vi "Behaviour Tree.vi"(10 "IO":T1) -> (3 "bt_Node out":refnum<class "bt_Node.lvclass">)   [LabVIEW 2021, in "Car Wash Support.lvlib"]
uses:
  Car Wash Support.lvlib
  IO Refs.ctl
  <vilib>/TSA/Abstract Data Classes/Abs_Types/Boolean/Abs_Boolean.lvclass
  <vilib>/TSA/Abstract Data Classes/Abs_Types/I32 Integer/Abs_I32 Integer.lvclass
  <vilib>/TSA/Abstract Data Classes/Abs_Types/Double Float/Abs_Double Float.lvclass
  <vilib>/TSA/Event Log/Event_TextLog/Event_TextLog.lvclass
  C:/Program Files (x86)/National Instruments/LabVIEW 2021/vi.lib/TSA/Event Log/abs_EventLog/abs_EventLog.lvclass
  Wash Indicators.ctl
  Wash Options.ctl
  Support/Nodes/abs_Node/bt_Node.lvclass
  Support/Nodes/Decorators/Repeater/Support/Finish On - Type.ctl
  Support/Nodes/Leaves/Log/bt_Log.lvclass
  C:/Users/timst/Documents/Repositories/LV_Behaviour_Tree/Source/Support/Nodes/abs_Node/bt_Node.lvclass
  <vilib>/TSA/Abstract Data Classes/Constants/Support/Str/Str.vi
  Support/Poly/Log/Log_StringClass.vi
  BT.lvlib
  Support/Nodes/Decorators/Repeater/bt_Repeater.lvclass
  <vilib>/TSA/Abstract Data Classes/Constants/Support/Str/Const_Str.lvclass
  C:/Program Files (x86)/National Instruments/LabVIEW 2021/vi.lib/TSA/Event Log/Event_TextLog/Event_TextLog.lvclass
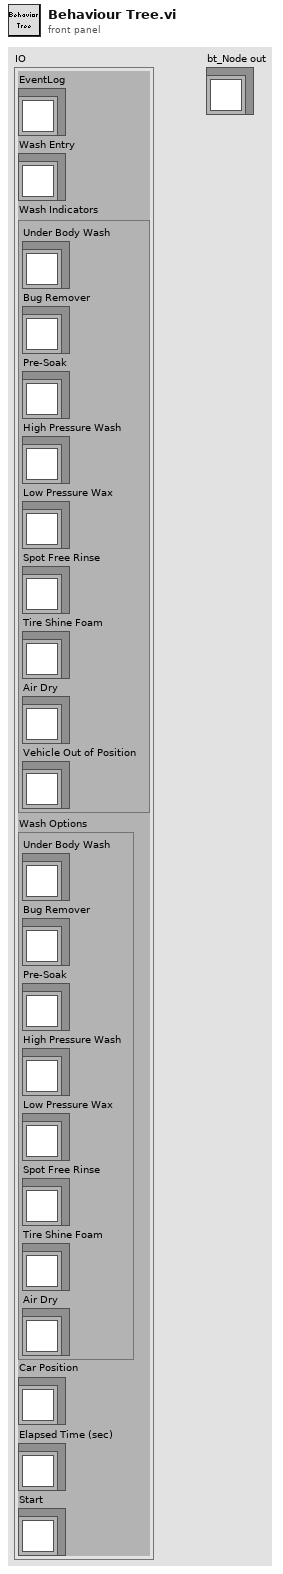
[diagram p1: front panel]
types:
  T1 = typedef "Car Wash Support.lvlib/IO Refs.ctl" = cluster{"EventLog":refnum<class "Event_TextLog.lvclass">, "Wash Entry":refnum<class "Abs_Boolean.lvclass">, "Wash Indicators":T2, "Wash Options":T3, "Car Position":refnum<class "Abs_I32 Integer.lvclass">, "Elapsed Time (sec)":refnum<class "Abs_Double Float.lvclass">, "Start":refnum<class "Abs_Boolean.lvclass">}
  T2 = typedef "Car Wash Support.lvlib/Wash Indicators.ctl" = cluster{"Under Body Wash":refnum<class "Abs_Boolean.lvclass">, "Bug Remover":refnum<class "Abs_Boolean.lvclass">, "Pre-Soak":refnum<class "Abs_Boolean.lvclass">, "High Pressure Wash":refnum<class "Abs_Boolean.lvclass">, "Low Pressure Wax":refnum<class "Abs_Boolean.lvclass">, "Spot Free Rinse":refnum<class "Abs_Boolean.lvclass">, "Tire Shine Foam":refnum<class "Abs_Boolean.lvclass">, "Air Dry":refnum<class "Abs_Boolean.lvclass">, "Vehicle Out of Position":refnum<class "Abs_Boolean.lvclass">}
  T3 = typedef "Car Wash Support.lvlib/Wash Options.ctl" = cluster{"Under Body Wash":refnum<class "Abs_Boolean.lvclass">, "Bug Remover":refnum<class "Abs_Boolean.lvclass">, "Pre-Soak":refnum<class "Abs_Boolean.lvclass">, "High Pressure Wash":refnum<class "Abs_Boolean.lvclass">, "Low Pressure Wax":refnum<class "Abs_Boolean.lvclass">, "Spot Free Rinse":refnum<class "Abs_Boolean.lvclass">, "Tire Shine Foam":refnum<class "Abs_Boolean.lvclass">, "Air Dry":refnum<class "Abs_Boolean.lvclass">}
  T4 = typedef "BT.lvlib/bt_Repeater.lvclass/Finish On - Type.ctl" = enum16{"Success", "Failure", "Never"}
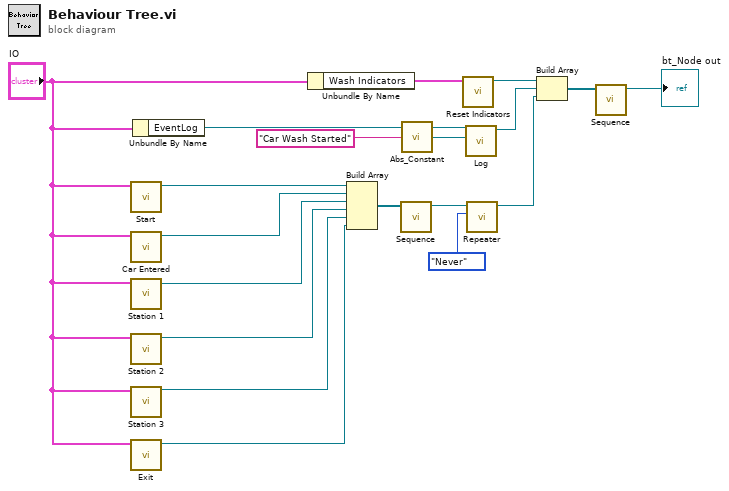
[diagram p0: block diagram]
diagram:
  n1 = call "Start.vi"("IO"="IO") -> ("bt_Node out"=w6:refnum<class "bt_Node.lvclass">)  [unwired: 10 in]
  n2 = call "Car Entered.vi"("IO"="IO") -> ("bt_Node out"=w5:refnum<class "bt_Node.lvclass">)  [unwired: 10 in]
  n3 = call "Station 1.vi"("IO"="IO") -> ("bt_Node out"=w1:refnum<class "bt_Node.lvclass">)  [unwired: 10 in]
  n4 = call "Station 2.vi"("IO"="IO") -> ("bt_Node out"=w4:refnum<class "bt_Node.lvclass">)  [unwired: 10 in]
  n5 = call "Station 3.vi"("IO"="IO") -> ("bt_Node out"=w3:refnum<class "bt_Node.lvclass">)  [unwired: 10 in]
  n6 = call "Exit.vi"("IO"="IO") -> ("bt_Node out"=w7:refnum<class "bt_Node.lvclass">)  [unwired: 10 in]
  n7 = Unbundle By Name("IO") -> ("EventLog"=w8:refnum<class "Event_TextLog.lvclass">)
  n8 = Unbundle By Name("IO") -> ("Wash Indicators"=w13:T2)
  n9 = Build Array(w6, w5, w1, w4, w3, w7) -> (w15:refnum<class "bt_Node.lvclass">[])
  n10 = call "Sequence.vi"("Nodes"=w15) -> ("Node"=w14:refnum<class "bt_Node.lvclass">)  [unwired: 10 in]
  n11 = call-poly <vilib>:"Abs_Constant.vi"("String"="Car Wash Started") -> ("Abs_String.lvclass"=w11:refnum<class "Abs_String.lvclass">)  [unwired: 4 in]
  n12 = call "Reset Indicators.vi"("Indicators"=w13) -> ("Node"=w12:refnum<class "bt_Node.lvclass">)  [unwired: 10 in]
  n13 = call-poly "Log.vi"("Message"=w11, "EventLog"=w8) -> ("node out"=w10:refnum<class "bt_Log.lvclass">)  [unwired: 9 in]
  n14 = call "Repeater.vi"("Finish On"=Finish_On_-_Type."Never", "Node In"=w14) -> ("Node Out"=w17:refnum<class "bt_Node.lvclass">)  [unwired: 9 in]
  n15 = Build Array(w12, w10, w17) -> (w18:refnum<class "bt_Node.lvclass">[])
  n16 = call "Sequence.vi"("Nodes"=w18) -> ("Node"=→"bt_Node out":refnum<class "bt_Node.lvclass">)  [unwired: 10 in]
